vi "Config.vi"(8 "error in (no error)":errorcluster, 10 "DMM Settings":T5={"Measurement Type"=enum."4-wire Resistance", "Offset Compensated Ohms"=1, "Resolution in Digits"=6.5, "Range"=100.0, "Auto Zero"=1} {"Auto Zero" items=["Auto"=-1, "Off"=0, "On"=1, "Once"=2]; "Range" format="%#_13g"; "Resolution in Digits" items=["3 1/2"=3.5, "4 1/2"=4.5, "5 1/2"=5.5, "6 1/2"=6.5, "7 1/2"=7.5]; "Offset Compensated Ohms" items=["Off", "On"]}, 11 "IVI Refnum in":refnum<k15>) -> (0 "error out":errorcluster, 3 "instrument handle out":refnum<k15>)   [LabVIEW 2013]
uses:
  <instrlib>/niDMM/nidmm.llb/niDMM Function.ctl
  <instrlib>/niDMM/nidmm.llb/niDMM Offset Comp Ohms.ctl
  <instrlib>/niDMM/nidmm.llb/niDMM Resolution in Digits.ctl
  <instrlib>/niDMM/nidmm.llb/niDMM Auto Zero.ctl
  <instrlib>/niDMM/nidmm.llb/niDMM Configure Measurement Digits.vi
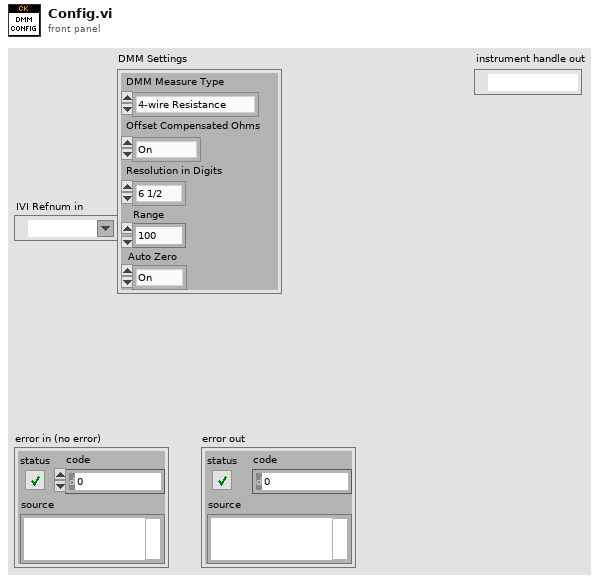
[diagram p1: front panel]
types:
  T1 = typedef "niDMM Function.ctl" = enum16{"DC Volts", "AC Volts", "DC Current", "AC Current", "2-wire Resistance", "4-wire Resistance", "Diode", "Frequency", "Period", "AC Volts DC Coupled", "Capacitance", "Inductance", "Temperature"}
  T2 = typedef "niDMM Offset Comp Ohms.ctl" = i32
  T3 = typedef "niDMM Resolution in Digits.ctl" = dbl
  T4 = typedef "niDMM Auto Zero.ctl" = i32
  T5 = cluster{"Measurement Type":T1, "Offset Compensated Ohms":T2, "Resolution in Digits":T3, "Range":dbl, "Auto Zero":T4}
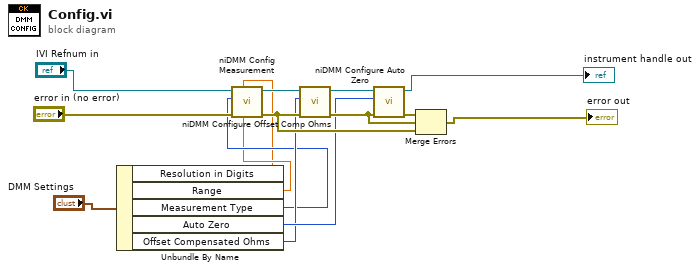
[diagram p0: block diagram]
diagram:
  n1 = Unbundle By Name("DMM Settings") -> ("Resolution in Digits"=w1:T3, "Range"=w2:dbl, "Measurement Type"=w3:T1, "Auto Zero"=w5:T4, "Offset Compensated Ohms"=w4:T2)
  n2 = call-poly <instrlib>:"niDMM Config Measurement.vi"("Range"=w2, "Resolution in Digits"=w1, "error in (no error)"="error in (no error)", "Function"=w3, "instrument handle"="IVI Refnum in") -> ("error out"=w15:errorcluster, "instrument handle out"=w10:refnum<k15>)  [unwired: 5 in]
  n3 = call <instrlib>:"niDMM Configure Offset Comp Ohms.vi"("error in (no error)"=w15, "Offset Compensated Ohms"=w4, "instrument handle"=w10) -> ("error out"=w14:errorcluster, "instrument handle out"=w11:refnum<k15>)  [unwired: 7 in]
  n4 = call <instrlib>:"niDMM Configure Auto Zero.vi"("error in (no error)"=w14, "Auto Zero"=w5, "instrument handle"=w11) -> ("error out"=w12:errorcluster, "instrument handle out"=→"instrument handle out":refnum<k15>)  [unwired: 7 in]
  n5 = Merge Errors(w12, w14, w15) -> (→"error out":errorcluster)
